vi "Get Kasli IP from Name.vi"(8 "error in (no error)":errorcluster, 10 "Kasli Name":string, 11 "Kasli in":refnum<class "Kasli.lvclass">) -> (0 "error out":errorcluster, 2 "IP":string, 3 "Kasli out":refnum<class "Kasli.lvclass">)   [LabVIEW 2020, in "TALOS.lvlib" / "Kasli Wrapper 2.0.lvlib" / "Kasli.lvclass"]
uses:
  Kasli.lvclass
  Kasli.lvclass/Kasli.ctl
  f74609e2-d7b5-4696-a2f7-77896b9945e1.vi
  f74609e2-d7b5-4696-a2f7-77896b9945e1.vi/d4db2432-cc9c-482c-8957-dac855435ef6.vi
  f74609e2-d7b5-4696-a2f7-77896b9945e1.vi/86fbf154-bd7b-49a2-8ab2-a837b2a95f24.vi
  f74609e2-d7b5-4696-a2f7-77896b9945e1.vi/3b95b01e-1ec2-4565-bcd9-7606a5281010.vi
  f74609e2-d7b5-4696-a2f7-77896b9945e1.vi/96a08935-737a-44b2-979c-a81d56408f7e.vi
  f74609e2-d7b5-4696-a2f7-77896b9945e1.vi/d4db2432-cc9c-482c-8957-dac855435ef6.vi/6eaecd13-6e48-4772-a921-b51ebdf84d88.vi
  f74609e2-d7b5-4696-a2f7-77896b9945e1.vi/d4db2432-cc9c-482c-8957-dac855435ef6.vi/d2d5f2b7-06f4-47f6-971c-049c3fdbb653.vi
  f74609e2-d7b5-4696-a2f7-77896b9945e1.vi/3b95b01e-1ec2-4565-bcd9-7606a5281010.vi/6eaecd13-6e48-4772-a921-b51ebdf84d88.vi
  f74609e2-d7b5-4696-a2f7-77896b9945e1.vi/3b95b01e-1ec2-4565-bcd9-7606a5281010.vi/d2d5f2b7-06f4-47f6-971c-049c3fdbb653.vi
  f74609e2-d7b5-4696-a2f7-77896b9945e1.vi/96a08935-737a-44b2-979c-a81d56408f7e.vi/6eaecd13-6e48-4772-a921-b51ebdf84d88.vi
  f74609e2-d7b5-4696-a2f7-77896b9945e1.vi/96a08935-737a-44b2-979c-a81d56408f7e.vi/d2d5f2b7-06f4-47f6-971c-049c3fdbb653.vi
  <vilib>/Comparison/Less/Less Functor/Less Functor.lvclass
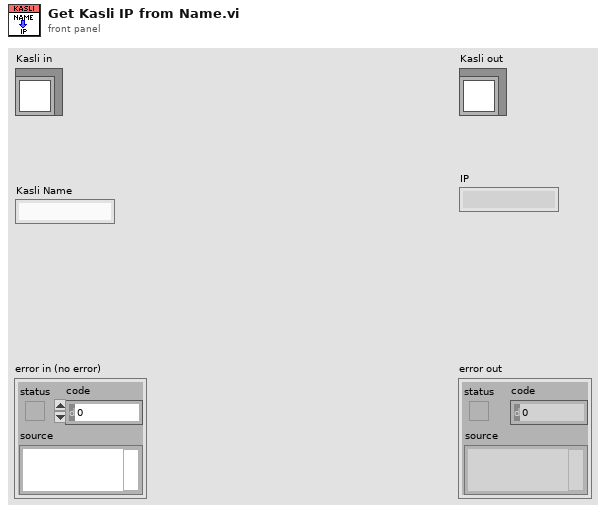
[diagram p1: front panel]
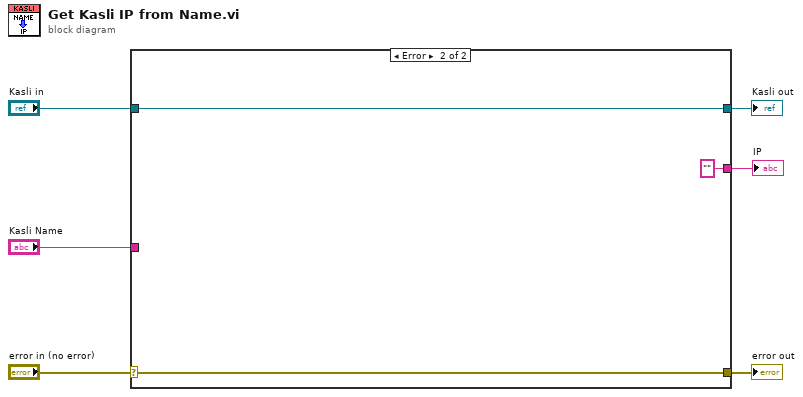
[diagram p0: block diagram]
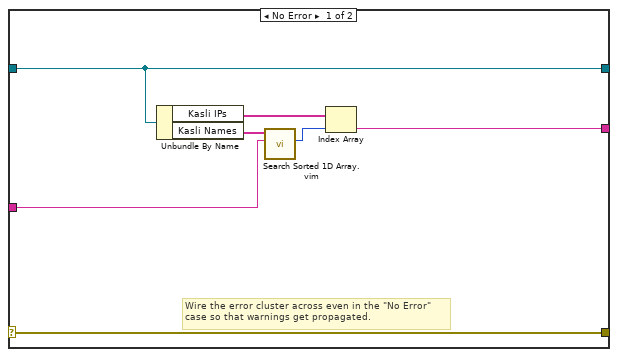
[diagram p2: hidden frame]
diagram:
  n1 = case shown="Error" "error in (no error)" {
    selector: "error in (no error)" -> [w13 w16]
    tunnel: [w13 w16] -> w5
    tunnel: [w12 w15] -> w3
    tunnel: "Kasli in" -> [w12 w15]
    tunnel: "Kasli Name" -> [w10 _]
    tunnel: [w7 "" ("IP")] -> w1
    frame No Error {
      # "Wire the error cluster across even in the \"No Error\"\ncase so that warnings get propagated."
      n2 = Unbundle By Name(w12) -> ("Kasli IPs"=w9:string[], "Kasli Names"=w11:string[])
      n3 = call "Search Sorted 1D Array.vim"("element"=w10, "sorted 1D array"=w11) -> ("nearest index"=w8:i32)  [unwired: 8 in, 1 out]
      n4 = Index Array(array=w9, index=w8) -> (element=w7:string)
    }
    frame Error {
    }
  }
  "error out" <- w5
  "Kasli out" <- w3
  "IP" <- w1
